vi "Check Firmware Version.vi"(8 "Error In":errorcluster, 11 "LINX Device Config":T1) -> (0 "Error Out":errorcluster, 3 "LINX Device Config":T1)   [LabVIEW 2011, in "LVH-LINX.lvlib" / "Device.lvlib"]
uses:
  Device.lvlib
  Type Defs/LINX Device Config.ctl
  Type Defs/Interface.ctl
  Type Defs/TCP Config.ctl
  Type Defs/Channels.ctl
  Type Defs/Error Type.ctl
  LVH-LINX.lvlib
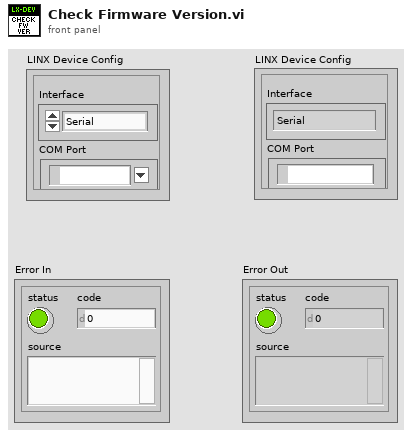
[diagram p1: front panel]
types:
  T1 = typedef "LVH-LINX.lvlib/Device.lvlib/LINX Device Config.ctl" = cluster{"Interface":T2, "COM Port":refnum<visa-resource-name>, "TCP Configuration":T3, "Device Family":u8, "Device ID":u8, "Device Name":string, "TCP Ref":refnum<k5>, "Channels":T4}
  T2 = typedef "LVH-LINX.lvlib/Interface.ctl" = enum16{"Serial", "TCP"}
  T3 = typedef "LVH-LINX.lvlib/Device.lvlib/TCP Config.ctl" = cluster{"IP Address":string, "Port":u16}
  T4 = typedef "LVH-LINX.lvlib/Channels.ctl" = cluster{"DI Channels":u8[], "DO Channels":u8[], "AI":u8[], "AO":u8[], "PWM":u8[], "QE":u8[], "UART":u8[], "I2C 2":u8[], "SPI":u8[], "CAN":u8[], "AI Ref (V)":dbl, "AO Resolution (Bits)":u8, "AO Ref (V)":dbl}
  T5 = typedef "LVH-LINX.lvlib/Device.lvlib/Firmware Version.ctl" = cluster{"Major":u8, "Minor":u8, "SubMinor":u8}
  T6 = typedef "LVH-LINX.lvlib/Error Type.ctl" = enum16{"Unknown", "Timeout", "Corrupt Return Packet", "Unable To Connect", "Command Not Supported", "Channel DNE", "Invalid COM Config", "Firmware Version Mismatch", "myRIO Support"}
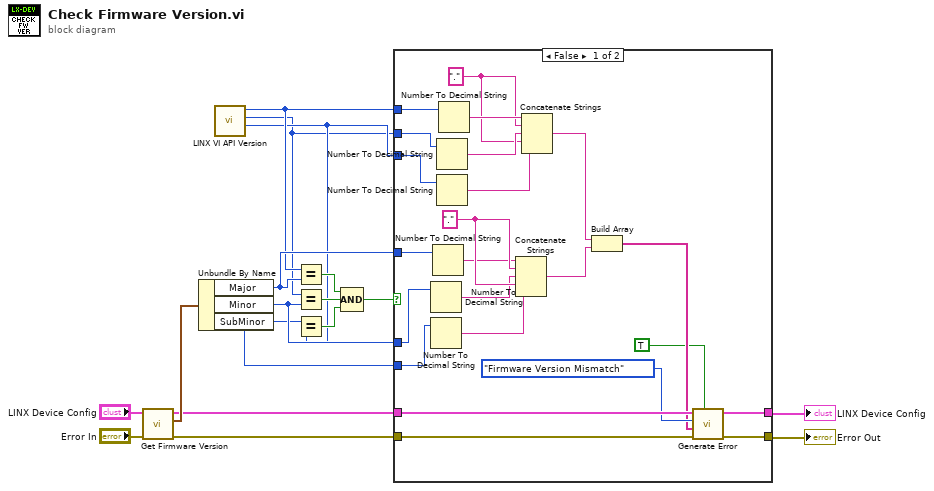
[diagram p0: block diagram]
diagram:
  n1 = call "Get Firmware Version.vi"("Error In"="Error In", "LINX Device Config"="LINX Device Config") -> ("Error Out"=w6:errorcluster, "LINX Firmware Version"=w15:T5, "LINX Device Config"=w7:T1)  [unwired: 7 in]
  n2 = Unbundle By Name(w15) -> ("Major"=w10:u8, "Minor"=w9:u8, "SubMinor"=w8:u8)
  n3 = call "LINX VI API Version.vi"() -> ("SubMinor"=w2:u8, "Minor"=w1:u8, "Major"=w3:u8)  [unwired: 9 in]
  n4 = Equal?(x=w3, y=w10) -> (x = y?=w12:bool)
  n5 = Equal?(x=w1, y=w9) -> (x = y?=w13:bool)
  n6 = Equal?(x=w8, y=w2) -> (x = y?=w14:bool)
  n7 = Compound Arithmetic op=AND(w12, w13, w14) -> (w11:bool)
  n8 = case shown="False" w11 {
    tunnel: w3 -> [w40 _]
    tunnel: w1 -> [w39 _]
    tunnel: w2 -> [w38 _]
    tunnel: w10 -> [w27 _]
    tunnel: w9 -> [w26 _]
    tunnel: w8 -> [w25 _]
    tunnel: w7 -> [w24 w42]
    tunnel: w6 -> [w23 w41]
    tunnel: [w20 w42] -> w5
    tunnel: [w19 w41] -> w4
    frame False {
      w32 = "." ("string")
      w35 = "." ("string")
      n9 = Number To Decimal String(number=w26) -> (decimal integer string=w31:string)  [unwired: 1 in]
      n10 = Number To Decimal String(number=w25) -> (decimal integer string=w33:string)  [unwired: 1 in]
      n11 = Number To Decimal String(number=w27) -> (decimal integer string=w30:string)  [unwired: 1 in]
      n12 = Number To Decimal String(number=w39) -> (decimal integer string=w36:string)  [unwired: 1 in]
      n13 = Number To Decimal String(number=w38) -> (decimal integer string=w34:string)  [unwired: 1 in]
      n14 = Number To Decimal String(number=w40) -> (decimal integer string=w37:string)  [unwired: 1 in]
      n15 = Concatenate Strings(w30, w32, w31, w32, w33) -> (w29:string)
      n16 = Concatenate Strings(w37, w35, w36, w35, w34) -> (w28:string)
      n17 = Build Array(w28, w29) -> (w21:string[])
      n18 = call "Generate Error.vi"("Is Warning? (False)"=TRUE, "Error In"=w23, "Arguments"=w21, "Error Type"=Error_Type."Firmware Version Mismatch", "LINX Device Config"=w24) -> ("Error Out"=w19:errorcluster, "LINX Device Config"=w20:T1)  [unwired: 5 in]
    }
    frame True {
      # "Firmware Match.  Continue"
    }
  }
  "Error Out" <- w4
  "LINX Device Config" <- w5
